vi "Read Winch Motor Config.vi"(8 "error in (no error)":errorcluster, 10 "Configuration In":variant, 11 "Climber in":refnum<class "Climber.lvclass">) -> (0 "error out":errorcluster, 3 "Climber out":refnum<class "Climber.lvclass">)   [LabVIEW 2019, in "Climber.lvlib" / "Climber.lvclass"]
uses:
  Climber.lvclass
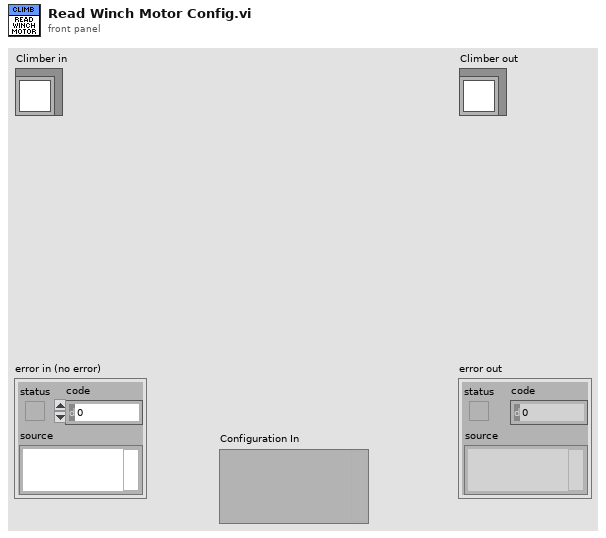
[diagram p1: front panel]
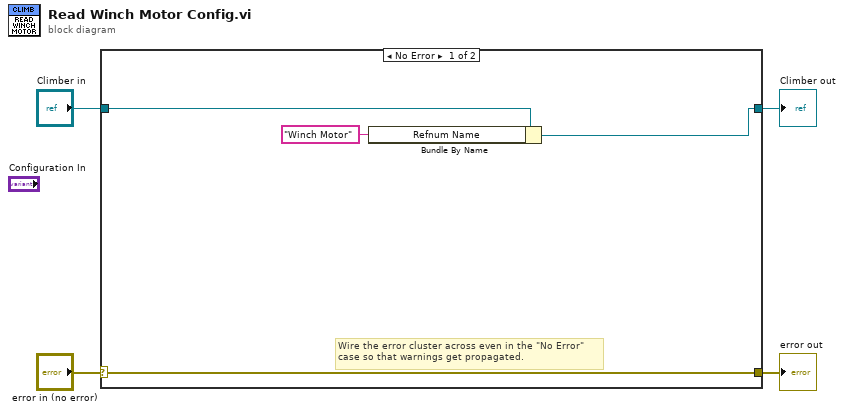
[diagram p0: block diagram]
diagram:
  n1 = case shown="No Error" "error in (no error)" {
    selector: "error in (no error)" -> [w8 w10]
    tunnel: [w8 w10] -> w3
    tunnel: [w5 w9] -> w1
    tunnel: "Climber in" -> [w7 w9]
    frame No Error {
      # "Wire the error cluster across even in the \"No Error\"\ncase so that warnings get propagated."
      n2 = Bundle By Name(cluster=w7, "Refnum Name"="Winch Motor" ("Winch Motor.Refnum Name")) -> (w5:refnum<class "Climber.lvclass">)
    }
    frame Error {
    }
  }
  "error out" <- w3
  "Climber out" <- w1
